vi "ShowIQvalues.vi"(11 "Waveform Graph":dbl[][](graph)) -> ()   [LabVIEW 2013]
panel:
  in  "OK Button":bool
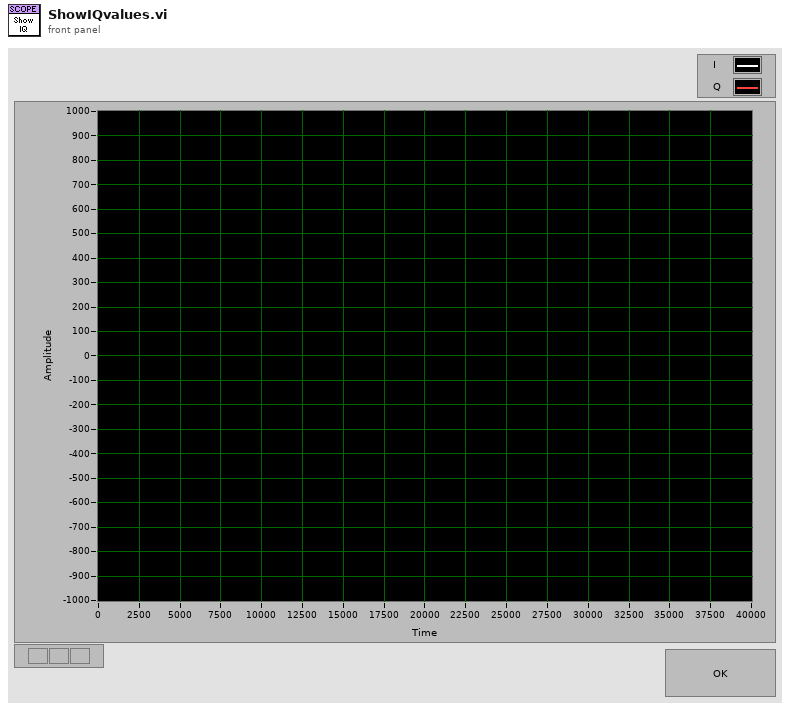
[diagram p1: front panel]
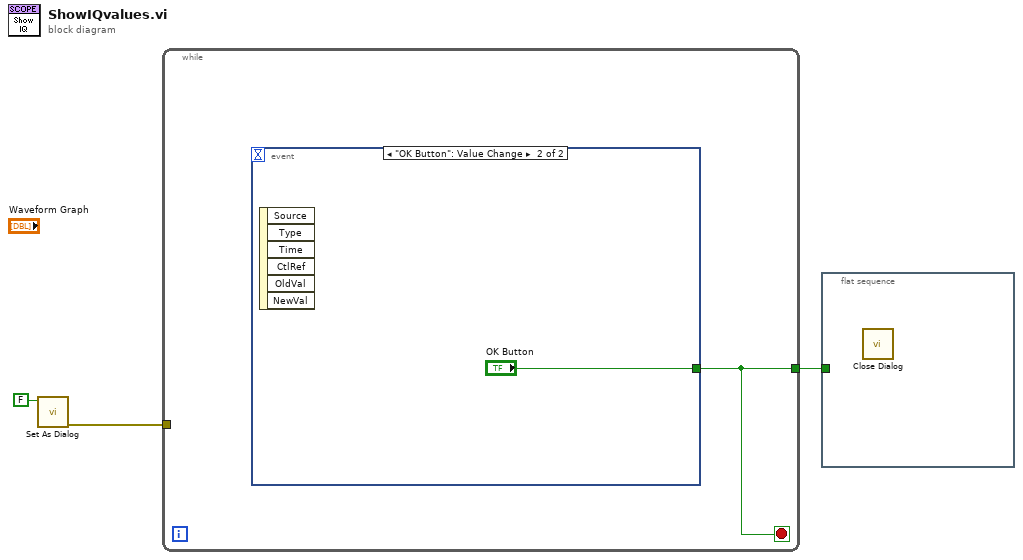
[diagram p0: block diagram]
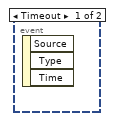
[diagram p2: hidden frame]
diagram:
  n1 = call "Set As Dialog.vi"("Only in RTE (T)"=FALSE) -> ("error out"=w3:errorcluster)  [unwired: 7 in]
  n2 = while {
    tunnel: w3 -> [_]
    tunnel: [w4] -> w1
    stop <- w4 stop-if-true
    n3 = event shown="[1] \"OK Button\": Value Change" {
      selector: _ -> [_ _]
      dyn-events: _ -> [_ _]
      timeout: _ -> [_ _]
      tunnel: [_ "OK Button"] -> w4
      event Timeout {
        n4 = event-data() -> ()  [unwired: 1 in, 3 out]
      }
      event "OK Button": Value Change {
        n5 = event-data() -> ()  [unwired: 1 in, 6 out]
      }
    }
  }
  n6 = flat-sequence {
    tunnel: w1 -> [_]
    frame #0 {
      n7 = call "Close Dialog.vi"() -> ()  [unwired: 8 in, 1 out]
    }
  }
